vi "Get Shown Card Map and Data.vi"(10 "Player":string, 11 "Hand Array":string[](array[string])) -> (1 "Total Hands":i32, 2 "Card Map":T1(array[cluster]), 3 "Shown Hands":string[](array[string]), 4 "Overall Profit Loss (BBs)":dbl)   [LabVIEW 2021]
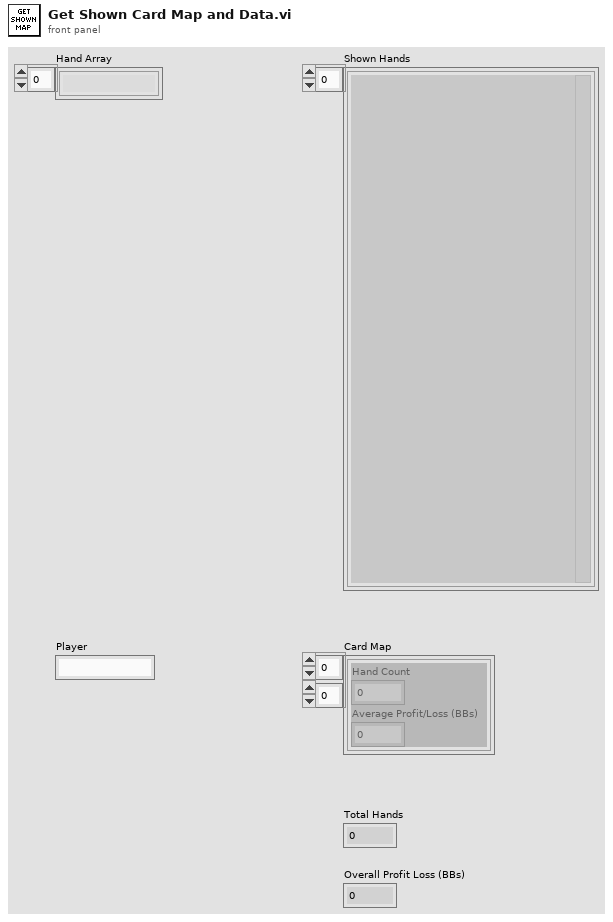
[diagram p1: front panel]
types:
  T1 = cluster{"Hand Count":u16, "Average Profit/Loss (BBs)":dbl}[][]
  T2 = cluster{"Hand Count":u16, "Average Profit/Loss (BBs)":dbl}
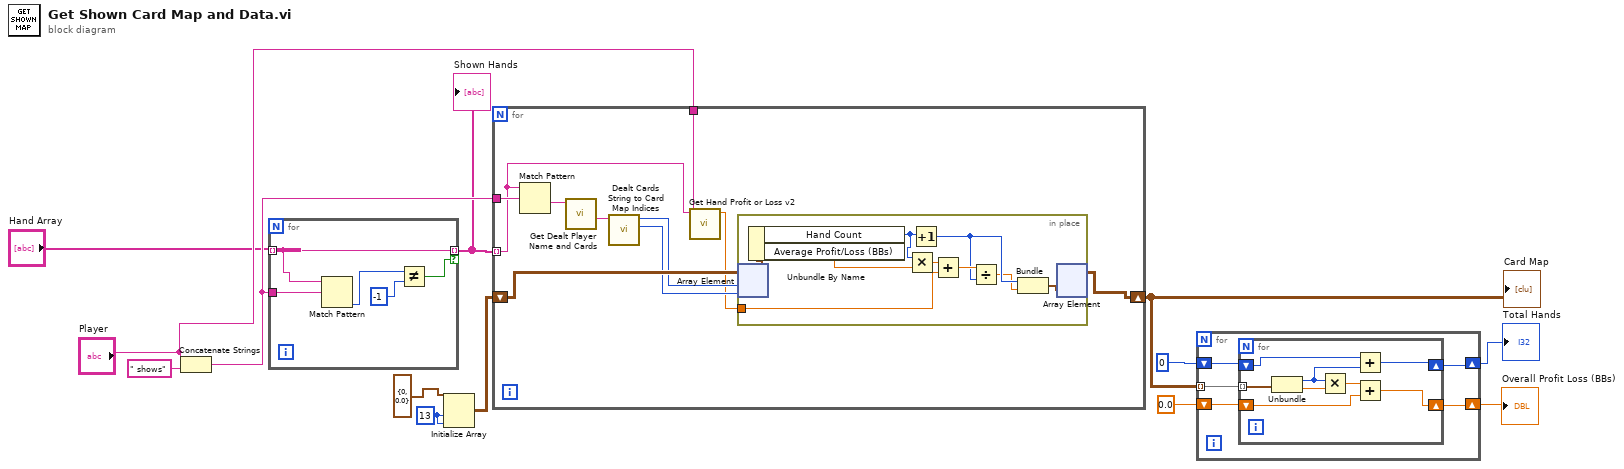
[diagram p0: block diagram]
diagram:
  w4 = 13 ("dimension size")
  n1 = Concatenate Strings("Player", " shows" ("string")) -> (w7:string)
  n2 = for {
    tunnel: "Hand Array" -> [w14] mode=indexing
    tunnel: w7 -> [w18]
    tunnel: [w14] -> w3 mode=indexing if=w17
    n3 = Match Pattern(string=w14, regular expression=w18) -> (offset past match=w16:i32)  [unwired: 1 in, 3 out]
    n4 = Not Equal?(x=w16, y=-1) -> (x != y?=w17:bool)
  }
  "Shown Hands" <- w3
  n5 = Initialize Array(T2 {"Hand Count"=0, "Average Profit/Loss (BBs)"=0.0} ("Cluster"), w4, w4) -> (w6:T1)
  n6 = for {
    tunnel: w3 -> [w26] mode=indexing
    shift-right: [w23] -> w11
    shift-left: w6 -> [w24]
    tunnel: w7 -> [w27]
    tunnel: "Player" -> [w25]
    n7 = Match Pattern(string=w26, regular expression=w27) -> (after substring=w28:string)  [unwired: 1 in, 3 out]
    n8 = call "Get Dealt Player Name and Cards.vi"("Hand History String in"=w28) -> ("Dealt Cards"=w22:string)  [unwired: 8 in, 2 out]
    n9 = call "Dealt Cards String to Card Map Indices.vi"("Dealt Cards String"=w22) -> ("Index1"=w20:i32, "Index0"=w21:i32)  [unwired: 9 in]
    n10 = call "Get Hand Profit or Loss v2.vi"("Dealt Player Name"=w25, "Hand History String"=w26) -> ("Profit/Loss (BBs)"=w19:dbl)  [unwired: 9 in]
    n11 = in-place {
      in-place-border: w19 -> [w36]
      n12 = in-place-array #1(w24, w21, w20) -> (w29:T2)
      n13 = Unbundle By Name(w29) -> ("Hand Count"=w31:u16, "Average Profit/Loss (BBs)"=w32:dbl)
      n14 = Multiply(x=w31, y=w32) -> (x*y=w37:dbl)
      n15 = Increment(x=w31) -> (x+1=w34:u16)
      n16 = Add(x=w37, y=w36) -> (x+y=w35:dbl)
      n17 = Divide(x=w35, y=w34) -> (x/y=w33:dbl)
      n18 = Bundle(w34, w33) -> (w30:cluster{u16, dbl})  [unwired: 1 in]
      n19 = in-place-array #1(w30) -> (w23:T1)  [unwired: 2 out]
    }
  }
  "Card Map" <- w11
  n20 = for {
    tunnel: w11 -> [w42] mode=indexing
    shift-right: [w40] -> w12
    shift-left: 0.0 -> [w41]
    shift-right: [w38] -> w13
    shift-left: 0 -> [w39]
    n21 = for {
      tunnel: w42 -> [w50] mode=indexing
      shift-right: [w46] -> w40
      shift-left: w41 -> [w47]
      shift-right: [w43] -> w38
      shift-left: w39 -> [w45]
      n22 = Unbundle(w50) -> ("Hand Count"=w44:u16, "Average Profit/Loss (BBs)"=w49:dbl)
      n23 = Multiply(x=w44, y=w49) -> (x*y=w48:dbl)
      n24 = Add(x=w45, y=w44) -> (x+y=w43:i32)
      n25 = Add(x=w48, y=w47) -> (x+y=w46:dbl)
    }
  }
  "Total Hands" <- w13
  "Overall Profit Loss (BBs)" <- w12
